vi "CloseFile.vi"(8 "error in (no error)":errorcluster, 11 "WOFile in":refnum<class "WOFile.lvclass">) -> (0 "error out":errorcluster)   [LabVIEW 2021, in "WOFile.lvclass"]
uses:
  WOFile.lvclass
  WOFile.lvclass/WOFile.ctl
  File/File.lvclass
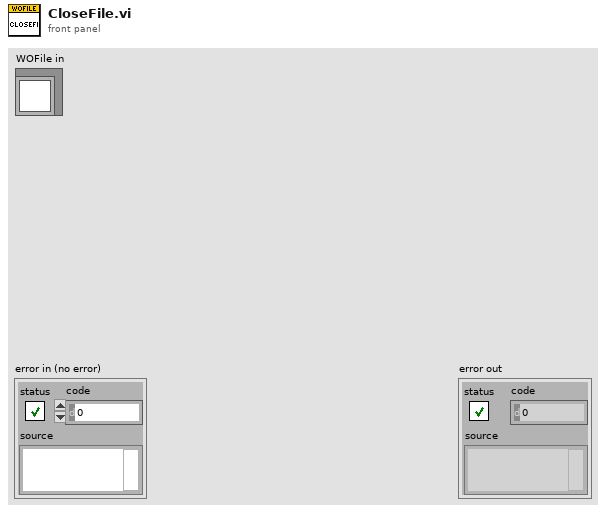
[diagram p1: front panel]
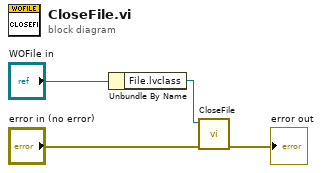
[diagram p0: block diagram]
diagram:
  n1 = Unbundle By Name("WOFile in") -> ("File.lvclass"=w1:refnum<class "File.lvclass">)
  n2 = call "CloseFile.vi"("error in (no error)"="error in (no error)", "File in"=w1) -> ("error out"=→"error out":errorcluster)  [unwired: 9 in]
